vi "KM101_SetParameter.vi"(6 "lVoltage":i32, 7 "lStepRate":i32, 8 "lStepAccn":i32, 9 "Channel":i32, 10 "reference in":refnum<k7>) -> (2 "reference out":refnum<k7>)   [LabVIEW 2018, in "KIM101lib.lvlib"]
uses:
  KIM101lib.lvlib
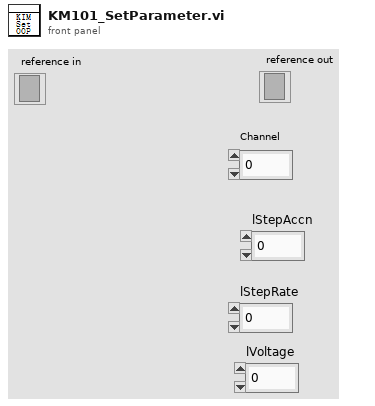
[diagram p1: front panel]
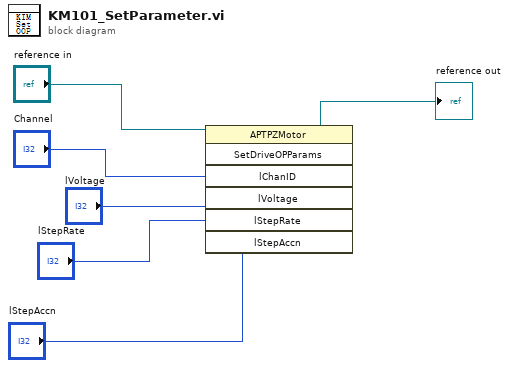
[diagram p0: block diagram]
diagram:
  n1 = invoke class="APTPZMotor" method="SetDriveOPParams"(reference="reference in", "lChanID"="Channel", "lVoltage"="lVoltage", "lStepRate"="lStepRate", "lStepAccn"="lStepAccn") -> (reference out=→"reference out":refnum<k7>)  [unwired: 2 in, 6 out]
